vi "OAT Torsional Vibration (Digital Tacho) (Even-Angle) (1 Ch).vi"(0 "digital tacho info":T3={"tacho counts"=[], "counter timebase [Hz]"=1000.0, "counter task type"=enum."event counting", "counter digit (32)"=32}, 2 "pulse/revolution (1)":i32=1 min=1, 4 "torsional vibration units":enum16{"RPM", "deg/s", "rad/s"}(ring), 5 "error in (no error)":errorcluster, 8 "reset? (F)":bool) -> (14 "even-angle torsional vibration signal":cluster{"r0":dbl, "dr":dbl, "Y":dbl[]}={"r0"=0.0, "dr"=1.0, "Y"=[]} {"r0" format="%.2p"; "dr" format="%.2p"; "Y" format="%.2f"}, 15 "even-angle channel info":T4={"channel name"="", "description"="", " channel info"={"sensor sensitivity"=1000.0, "engineering units"=1, "dB reference"=1.0, "custom label"="EU", "weighting filter"=0, "pregain"=0.0}} {"channel info"."pregain" format="%.2f"; "channel info"."weighting filter" items=["Linear", "A-weighting", "B-weighting", "C-weighting", "ITU-R 468-4", "Dolby", "CCITT", "C-message", "Wb", "Wc", "Wd", "We", "Wf", "Wh", "Wj", "Wk", "Wm", "AES17 20 kHz lowpass", "AES17 40 kHz lowpass", "AES17 20 kHz highpass", "AES17 40 kHz highpass"]; "channel info"."dB reference" format="%^.1e"; "channel info"."engineering units" items=["custom..."=0, "V"=1, "A"=21, "C"=30, "pC"=31, "s"=32, "-"=29, "Pa"=2, "N"=20, "g"=3, "m/s^2"=4, "m/s"=5, "m"=6, "mm/s"=12, "mm"=13, "micron/s"=14, "micron"=15, "in/s^2"=7, "in/s"=8, "in"=9, "mil/s"=10, "mil"=11, "rad/s^2"=16, "rad/s"=17, "rad"=18, "deg/s^2"=26, "deg/s"=27, "deg"=28, "RPM"=22, "cycle/s^2"=23, "Hz"=24, "cycle"=25, "strain"=19]; "channel info"."sensor sensitivity" format="%#_5f"}, 16 "speed profile":T2 {"speed [RPM]" format="%.2f"; "time [s]" format="%.2f"}, 17 "position info":T1, 18 "unit label":string, 19 "error out":errorcluster)   [LabVIEW 2017, in "SoundVib_Torsional.lvlib"]
doc: "Calculates torsional vibration signals from digital tachometer signals. This VI can return torsional vibration signals as either waveform signals or even-angle signals. Wire data to the <B>digital tacho info</B> input to determine the polymorphic instance to use or manually select the instance."
uses:
  <vilib>/addons/Sound and Vibration/Order Analysis/Torsional Vibration/SoundVib_Torsional.lvlib
  <vilib>/addons/_NISVFA/_Shared subVIs/Controls/svc_Resampled Channel Info.ctl
  <vilib>/addons/_NISVFA/_Shared subVIs/Controls/svc_Channel Info.ctl
  <vilib>/addons/_NISVFA/_Shared subVIs/Controls/svc_Engineering Units Text Ring.ctl
  <vilib>/addons/_NISVFA/_Shared subVIs/Controls/svc_Weighting Filter Text Ring.ctl
  <vilib>/addons/Sound and Vibration/Order Analysis/Tach Process/SubVIs/digital tach info.ctl
  <vilib>/addons/Sound and Vibration/Order Analysis/Tach Process/SubVIs/speed profile.ctl
  <vilib>/addons/Sound and Vibration/Order Analysis/Misc/OAT Position Info.ctl
  <vilib>/addons/Sound and Vibration/Order Analysis/Tach Process/SoundVib_TachProcess.lvlib
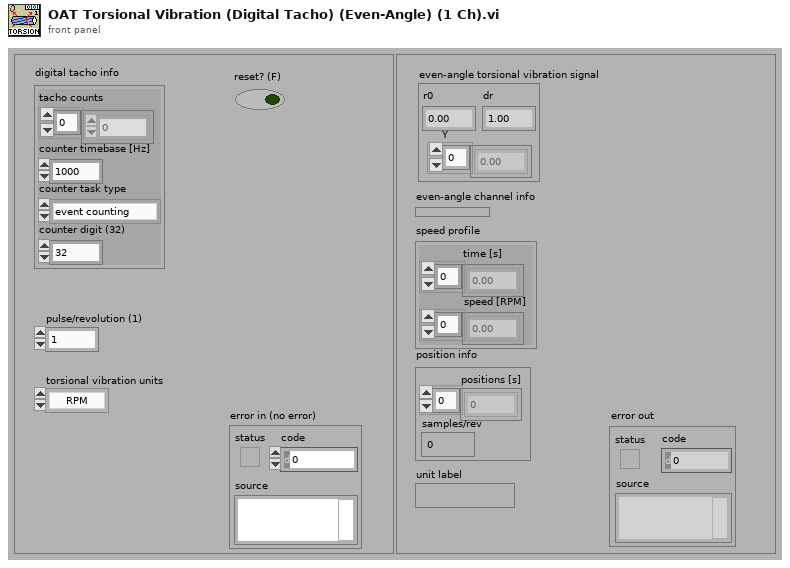
[diagram p1: front panel]
types:
  T1 = typedef "OAT Position Info.ctl" = cluster{"positions [s]":dbl[], "samples/rev":dbl}
  T2 = typedef "SoundVib_TachProcess.lvlib/speed profile.ctl" = cluster{"time [s]":dbl[], "speed [RPM]":dbl[]}
  T3 = typedef "SoundVib_TachProcess.lvlib/digital tach info.ctl" = cluster{"tacho counts":i64[], "counter timebase [Hz]":dbl, "counter task type":enum16{"period measurement", "event counting"}, "counter digit (32)":i32}
  T4 = typedef "svc_Resampled Channel Info.ctl" = cluster{"channel name":string, "description":string, " channel info":T5}
  T5 = typedef "svc_Channel Info.ctl" = cluster{"sensor sensitivity":dbl, "engineering units":T6, "dB reference":dbl, "custom label":string, "weighting filter":T7, "pregain":dbl}
  T6 = typedef "svc_Engineering Units Text Ring.ctl" = u16
  T7 = typedef "svc_Weighting Filter Text Ring.ctl" = u16
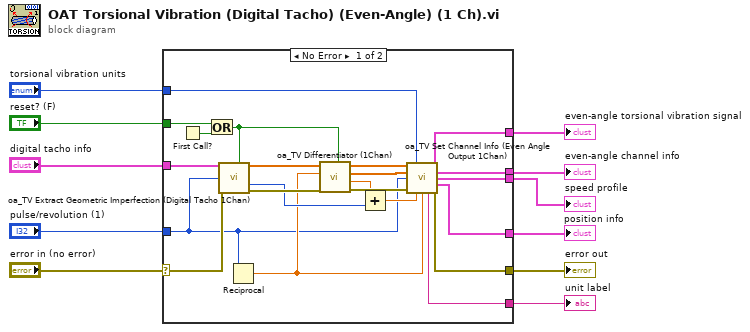
[diagram p0: block diagram]
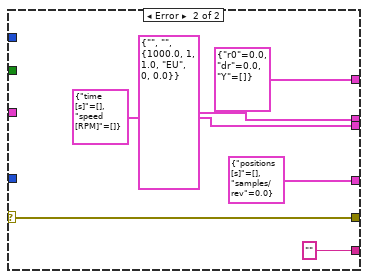
[diagram p2: hidden frame]
diagram:
  n1 = case shown="No Error" "error in (no error)" {
    selector: "error in (no error)" -> [w27 w39]
    tunnel: "pulse/revolution (1)" -> [w15 _]
    tunnel: [w21 cluster{"r0":dbl, "dr":dbl, "Y":dbl[]} {"r0"=0.0, "dr"=0.0, "Y"=[]} ("even-angle torsional vibration")] -> w7
    tunnel: "reset? (F)" -> [w30 _]
    tunnel: "digital tacho info" -> [w29 _]
    tunnel: "torsional vibration units" -> [w19 _]
    tunnel: [w25 w39] -> w8
    tunnel: [w22 T4 {"channel name"="", "description"="", " channel info"={"sensor sensitivity"=1000.0, "engineering units"=1, "dB reference"=1.0, "custom label"="EU", "weighting filter"=0, "pregain"=0.0}} ("even-angle channel info")] -> w6
    tunnel: [w17 "" ("unit label")] -> w3
    tunnel: [w14 T2 {"time [s]"=[], "speed [RPM]"=[]} ("speed profile")] -> w2
    tunnel: [w13 T1 {"positions [s]"=[], "samples/rev"=0.0} ("position info")] -> w1
    frame No Error {
      n2 = First Call?() -> (First Call?: T/F=w31:bool)
      n3 = Or(x=w30, y=w31) -> (x .or. y?=w18:bool)
      n4 = call <vilib>:"oa_TV Extract Geometric Imperfection (Digital Tacho 1Chan).vi"("digital tach info"=w29, "reset? (F)"=w18, "pulse/revolution"=w15, "error in (no error)"=w27) -> ("pulse positions"=w28:dbl[], "revulotion index"=w32:i32, "error out"=w33:errorcluster)  [unwired: 8 in, 1 out]
      n5 = Reciprocal(x=w15) -> (1/x=w23:dbl)
      n6 = call <vilib>:"oa_TV Differentiator (1Chan).vi"("reset? (True)"=w18, "error in (no error)"=w33, "deltaX"=w23, "Y[n]"=w28) -> ("error out"=w26:errorcluster, "Delay"=w12:dbl, "X[n]"=w16:dbl[], "dY[n]/dX[n]"=w20:dbl[])  [unwired: 4 in]
      n7 = Add(x=w12, y=w32) -> (x+y=w24:dbl)
      n8 = call <vilib>:"oa_TV Set Channel Info (Even Angle Output 1Chan).vi"("seconds/rev"=w20, "torisional vibration unit (RPM)"=w19, "pulse position"=w16, "pulse/revolution (1)"=w15, "error in (no error)"=w26, "r0"=w24, "dr"=w23) -> ("even-angle torsional vibration"=w21:cluster{"r0":dbl, "dr":dbl, "Y":dbl[]}, "even-angle channel info"=w22:T4, "speed profile"=w14:T2, "position info"=w13:T1, "unit label"=w17:string, "error out"=w25:errorcluster)  [unwired: 3 in]
    }
    frame Error {
    }
  }
  "error out" <- w8
  "even-angle channel info" <- w6
  "even-angle torsional vibration signal" <- w7
  "unit label" <- w3
  "position info" <- w1
  "speed profile" <- w2
